vi "Set MICS ID.vi"(4 "error in":errorcluster, 6 "MICS_ID":u32 format="%06x") -> (0 "error out":errorcluster)   [LabVIEW 2010]
uses:
  MICS_ID Global.vi
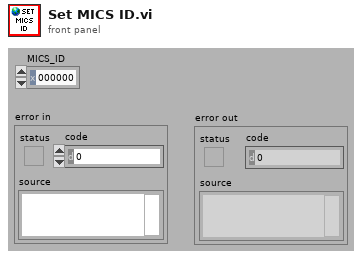
[diagram p1: front panel]
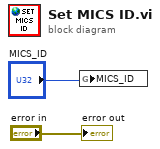
[diagram p0: block diagram]
diagram:
  n1 = global write "MICS_ID Global.vi" "MICS_ID"("MICS_ID") -> ()
  "error out" <- "error in"
